vi "Send Device Activate.vi"(6 "Activate Mode":T1, 7 "Message Priority (Normal)":T2=enum."Normal", 8 "error in (no error)":errorcluster, 10 "IED Name":string, 11 "Message Enqueuer":refnum<class "Message Enqueuer.lvclass">) -> (0 "error out":errorcluster, 3 "Message Enqueuer out":refnum<class "Message Enqueuer.lvclass">)   [LabVIEW 2015, in "SCADA Core.lvlib" / "Device Activate Msg.lvclass"]
doc: "This VI sends the message to an actor."
uses:
  Device Activate Msg.lvclass
  <vilib>/ActorFramework/Message Enqueuer/Message Enqueuer.lvclass
  <vilib>/ActorFramework/Message Enqueuer/Message Priority.ctl
  IED Actor/IED/Controls/Device Activate Mode Select.ctl
  Device Activate Msg.lvclass/Device Activate Msg.ctl
  <vilib>/ActorFramework/Message Enqueuer/Message Enqueuer.lvclass/Message Enqueuer.ctl
  <vilib>/ActorFramework/Message Priority Queue/Priority Enqueue.vi
  IED Actor/IED/IED.lvclass
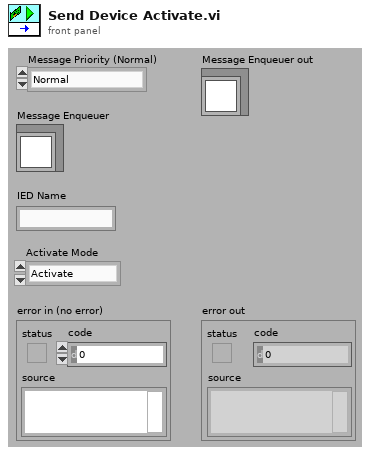
[diagram p1: front panel]
types:
  T1 = typedef "IED Actor.lvlib/IED.lvclass/Device Activate Mode Select.ctl" = enum16{"Activate", "Blackstart", "Individual"}
  T2 = typedef "Actor Framework.lvlib/Message Enqueuer.lvclass/Message Priority.ctl" = enum16{"Low", "Normal", "High"}
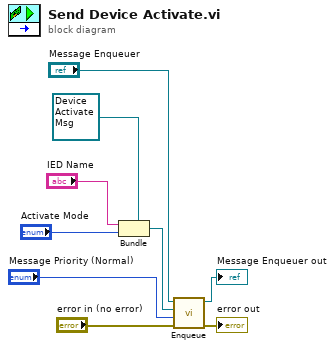
[diagram p0: block diagram]
diagram:
  n1 = Bundle(cluster=refnum<class "Device Activate Msg.lvclass"> refnum ("Object"), "IED Name", "Activate Mode") -> (w5:refnum<class "Device Activate Msg.lvclass">)
  n2 = call <vilib>:"Enqueue.vi"("error in (no error)"="error in (no error)", "Message Priority (Normal)"="Message Priority (Normal)", "Message"=w5, "Message Enqueuer in"="Message Enqueuer") -> ("error out"=→"error out":errorcluster, "Message Enqueuer out"=→"Message Enqueuer out":refnum<class "Message Enqueuer.lvclass">)  [unwired: 6 in]
